vi "EmergencyPowerStateController.vi"(1 "Master State":string) -> ()   [LabVIEW 2019]
doc: "This VI decides whether or not power should be diverted away from non-critical subsystems in an emergency or during certain periods of the match."
uses:
  outputs.vi
  sensors.vi
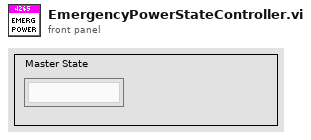
[diagram p1: front panel]
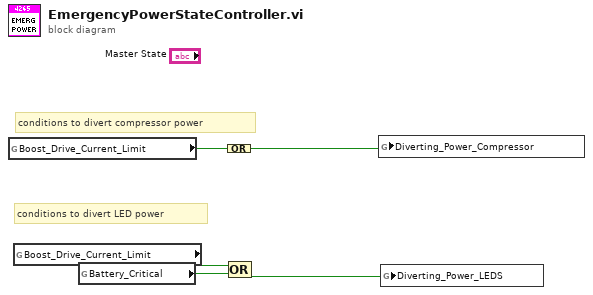
[diagram p0: block diagram]
diagram:
  # "conditions to divert LED power"
  # "conditions to divert compressor power"
  n1 = global read "outputs.vi" "Boost_Drive_Current_Limit"() -> (w4:bool)
  n2 = global read "outputs.vi" "Boost_Drive_Current_Limit"() -> (w2:bool)
  n3 = global read "sensors.vi" "Battery_Critical"() -> (w1:bool)
  n4 = Compound Arithmetic op=OR(w4) -> (w5:bool)
  n5 = Compound Arithmetic op=OR(w2, w1) -> (w3:bool)
  n6 = global write "outputs.vi" "Diverting_Power_Compressor"(w5) -> ()
  n7 = global write "outputs.vi" "Diverting_Power_LEDS"(w3) -> ()
